vi "Axe_card.vi"(7 "Operate Axis":T1(radio), 8 "error in (no error)":errorcluster, 9 "Servo On":bool, 10 "CFG_AxJogPAssign":u32, 11 "Function":T2(ring)) -> (0 "error out":errorcluster, 1 "Axis State:":string, 2 "Position":dbl, 3 "JOGSuccess":bool)   [LabVIEW 2016]
panel:
  out "ORG":bool
  out "EZ":bool
  out "HLMT+":bool
  out "HLMT-":bool
  in  "JDec":dbl=10000.0
  in  "JAcc":dbl=10000.0
  in  "JVelL":dbl=10000.0
  in  "JVelH":dbl=10000.0
  in  "JVLTime":u32=10000
  out "Servo_Off":bool
  out "Servo_On":bool
  out "CloseSuccess":bool
  out "ResetCounter":bool
  out "StopExtDriveSuccess":bool
  out "DeviceOpened":bool
  out "AxisOpened":bool
  out "AxisHandle_Array":u32[](array[numeric])
  out "DevAxesCount":u32
  out "DeviceHandle":u32
  in  "Device Type":u16(ring)
  out "DeviceNum List":u32[](array[numeric])
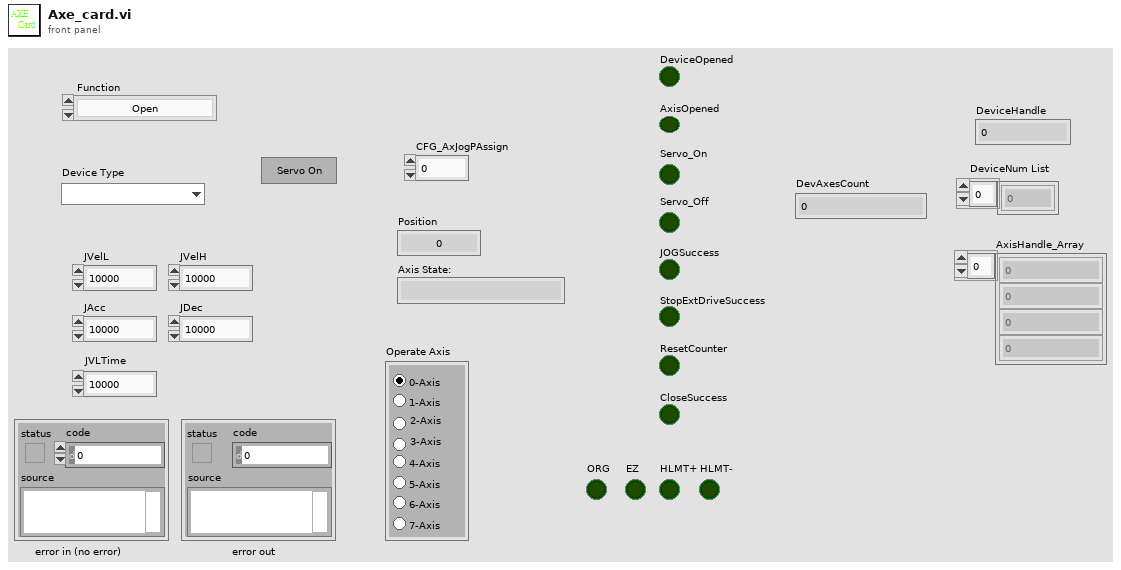
[diagram p1: front panel]
types:
  T1 = enum32{"0-Axis", "1-Axis", "2-Axis", "3-Axis", "4-Axis", "5-Axis", "6-Axis", "7-Axis"}
  T2 = enum16{"Open", "Move", "Check done", "E.Stop", "Get posion", "Home", "Serv ON/OFF", "Reset Error", "Set Param", "Close"}
  T3 = enum32{"CFG_AxJogVLTime", "CFG_AxPulseOutReverse", "CFG_AxKillDec", "CFG_AxJogVelLow", "CFG_AxJogVelHigh", "CFG_AxJogAcc", "CFG_AxJogDec", "CFG_AxJogJerk", "CFG_AxMaxErrorCnt", "CFG_AxCounterMax", "CFG_AxOverflowMode", "CFG_AxGantryActDiffValue", "CFG_AxJogPAssign", "CFG_AxJogNAssign", "CFG_AxCamDOAssign", "CFG_AxIN1StopAssign"}
  T4 = cluster{"DeviceNum":u32, "U*8 Array":cluster{"U*8 Array[0]":u8, "U*8 Array[1]":u8, "U*8 Array[2]":u8, "U*8 Array[3]":u8, "U*8 Array[4]":u8, "U*8 Array[5]":u8, "U*8 Array[6]":u8, "U*8 Array[7]":u8, "U*8 Array[8]":u8, "U*8 Array[9]":u8, "U*8 Array[10]":u8, "U*8 Array[11]":u8, "U*8 Array[12]":u8, "U*8 Array[13]":u8, "U*8 Array[14]":u8, "U*8 Array[15]":u8, "U*8 Array[16]":u8, "U*8 Array[17]":u8, "U*8 Array[18]":u8, "U*8 Array[19]":u8, "U*8 Array[20]":u8, "U*8 Array[21]":u8, "U*8 Array[22]":u8, "U*8 Array[23]":u8, "U*8 Array[24]":u8, "U*8 Array[25]":u8, "U*8 Array[26]":u8, "U*8 Array[27]":u8, "U*8 Array[28]":u8, "U*8 Array[29]":u8, "U*8 Array[30]":u8, "U*8 Array[31]":u8, "U*8 Array[32]":u8, "U*8 Array[33]":u8, "U*8 Array[34]":u8, "U*8 Array[35]":u8, "U*8 Array[36]":u8, "U*8 Array[37]":u8, "U*8 Array[38]":u8, "U*8 Array[39]":u8, "U*8 Array[40]":u8, "U*8 Array[41]":u8, "U*8 Array[42]":u8, "U*8 Array[43]":u8, "U*8 Array[44]":u8, "U*8 Array[45]":u8, "U*8 Array[46]":u8, "U*8 Array[47]":u8, "U*8 Array[48]":u8, "U*8 Array[49]":u8}, "NumOfSubDevice":i16}[]
  T5 = cluster{"U*8 Array[0]":u8, "U*8 Array[1]":u8, "U*8 Array[2]":u8, "U*8 Array[3]":u8, "U*8 Array[4]":u8, "U*8 Array[5]":u8, "U*8 Array[6]":u8, "U*8 Array[7]":u8, "U*8 Array[8]":u8, "U*8 Array[9]":u8, "U*8 Array[10]":u8, "U*8 Array[11]":u8, "U*8 Array[12]":u8, "U*8 Array[13]":u8, "U*8 Array[14]":u8, "U*8 Array[15]":u8, "U*8 Array[16]":u8, "U*8 Array[17]":u8, "U*8 Array[18]":u8, "U*8 Array[19]":u8, "U*8 Array[20]":u8, "U*8 Array[21]":u8, "U*8 Array[22]":u8, "U*8 Array[23]":u8, "U*8 Array[24]":u8, "U*8 Array[25]":u8, "U*8 Array[26]":u8, "U*8 Array[27]":u8, "U*8 Array[28]":u8, "U*8 Array[29]":u8, "U*8 Array[30]":u8, "U*8 Array[31]":u8, "U*8 Array[32]":u8, "U*8 Array[33]":u8, "U*8 Array[34]":u8, "U*8 Array[35]":u8, "U*8 Array[36]":u8, "U*8 Array[37]":u8, "U*8 Array[38]":u8, "U*8 Array[39]":u8, "U*8 Array[40]":u8, "U*8 Array[41]":u8, "U*8 Array[42]":u8, "U*8 Array[43]":u8, "U*8 Array[44]":u8, "U*8 Array[45]":u8, "U*8 Array[46]":u8, "U*8 Array[47]":u8, "U*8 Array[48]":u8, "U*8 Array[49]":u8}
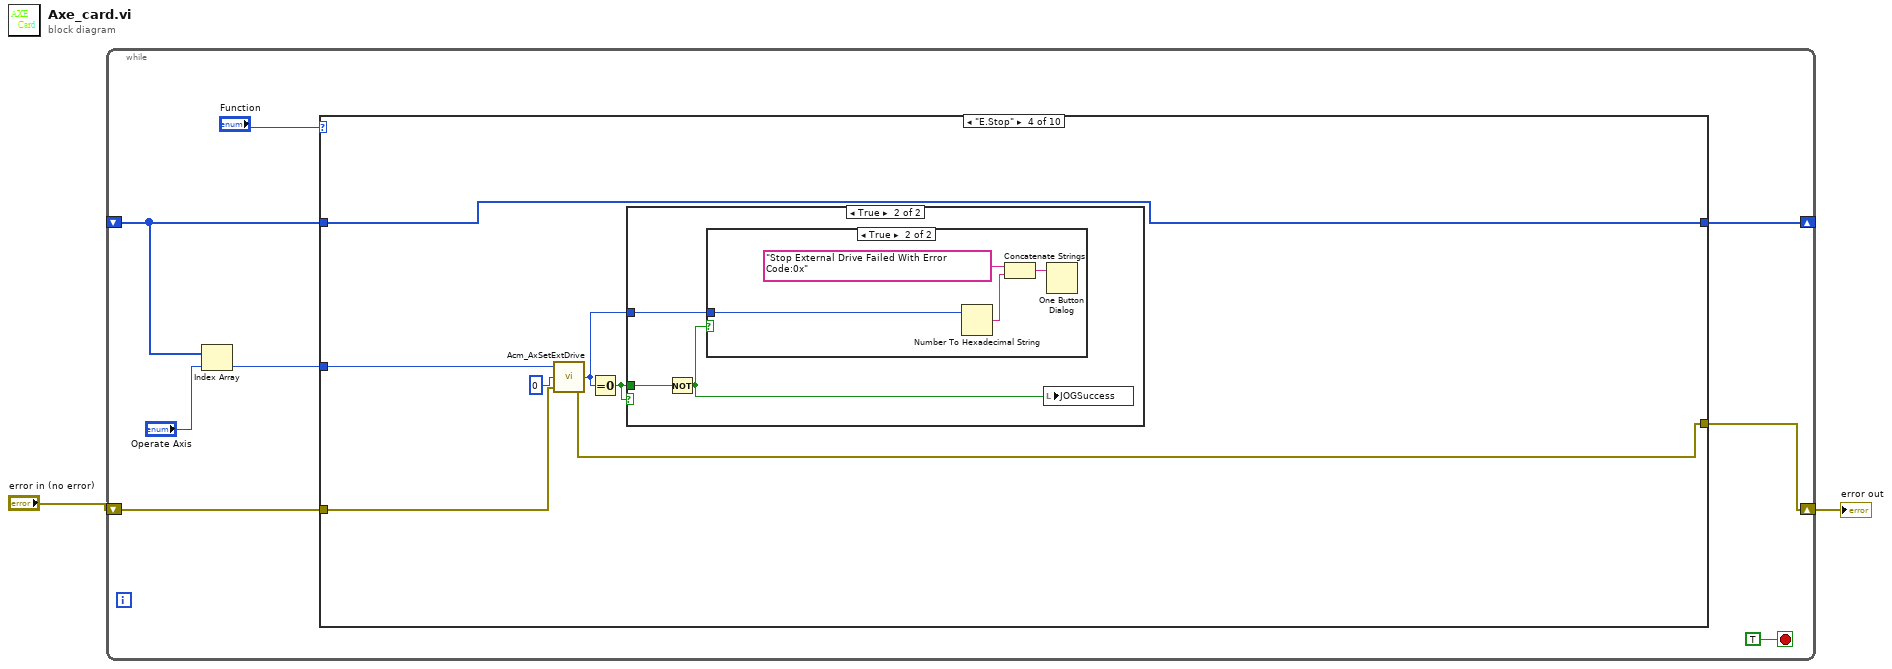
[diagram p0: block diagram]
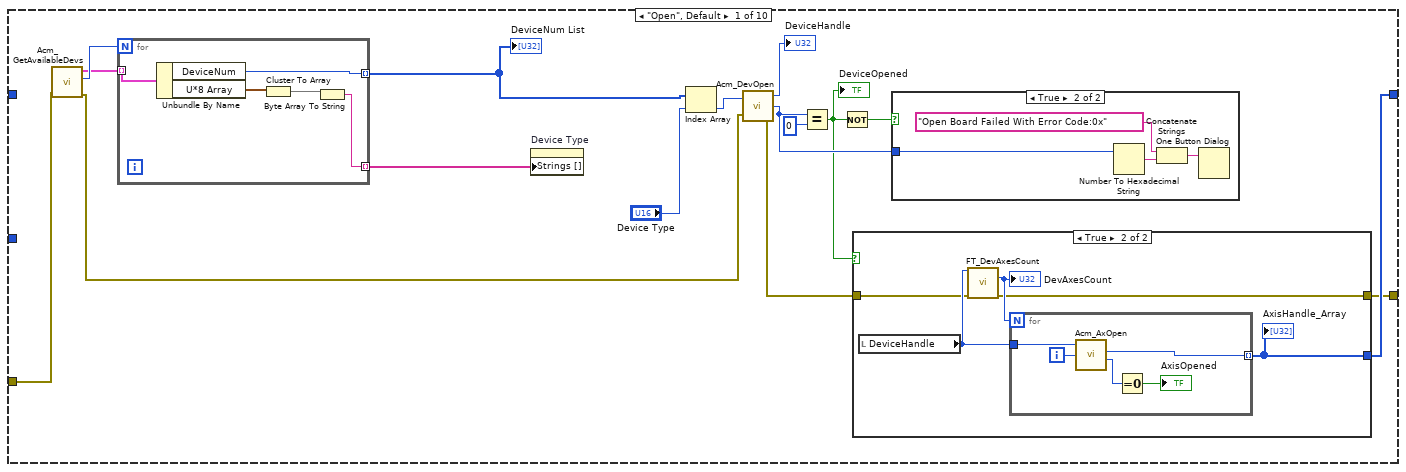
[diagram p2: hidden frame]
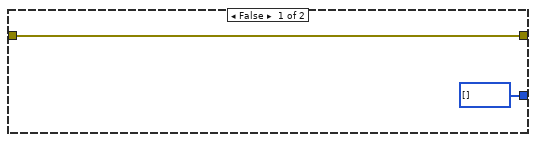
[diagram p4: hidden frame]
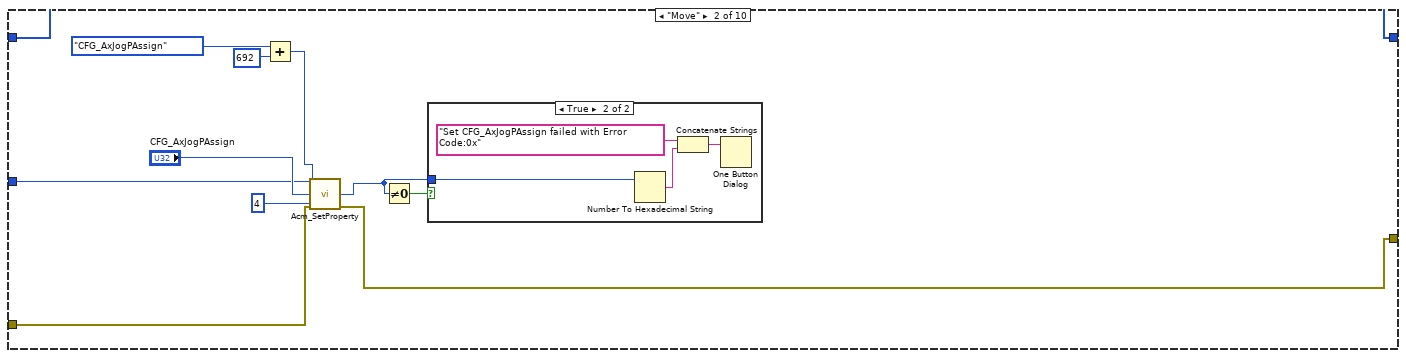
[diagram p5: hidden frame]
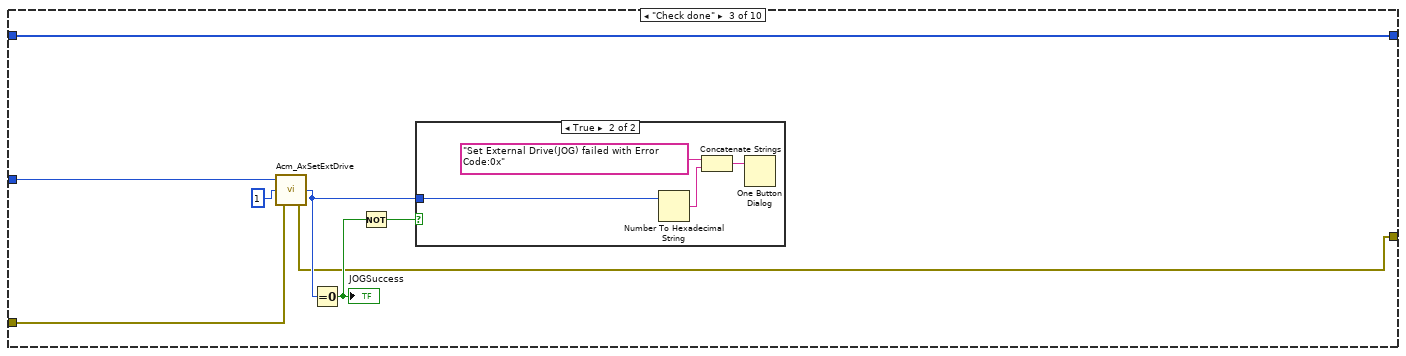
[diagram p7: hidden frame]
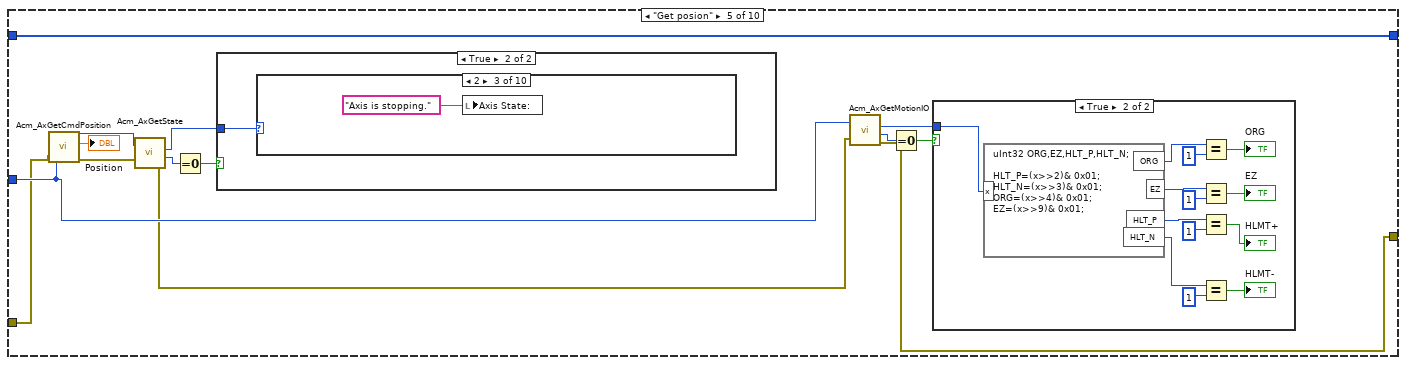
[diagram p11: hidden frame]
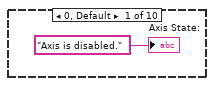
[diagram p14: hidden frame]
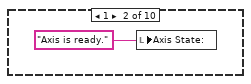
[diagram p15: hidden frame]
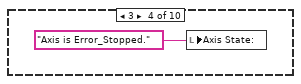
[diagram p16: hidden frame]
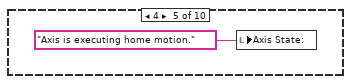
[diagram p17: hidden frame]
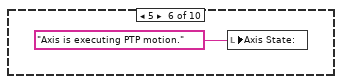
[diagram p18: hidden frame]
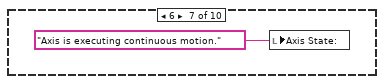
[diagram p19: hidden frame]
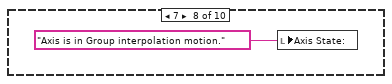
[diagram p20: hidden frame]
diagram:
  n1 = while {
    shift-right: [w8] -> _
    shift-left: _ -> [w7]
    shift-right: [w3] -> w1
    shift-left: "error in (no error)" -> [w4]
    stop <- TRUE stop-if-true
    n2 = Index Array(array=w7, index="Operate Axis") -> (element=w6:u32)
    n3 = case shown="\"E.Stop\"" "Function" {
      tunnel: [w16 w50 w65 w77 w97 w128 w149 w167 w176 w242] -> w8
      tunnel: w7 -> [_ w50 w65 w77 w97 w128 w149 w167 w176 w242]
      tunnel: w6 -> [_ w51 w66 w78 w93 w131 w151 w168 w177 _]
      tunnel: w4 -> [w14 w49 w64 w76 w92 w127 w145 w166 w175 w241]
      tunnel: [w11 w48 w63 w75 w89 w126 w144 w165 w174 w240] -> w3
      frame "Open", Default {
        n4 = call <userlib>:"Acm_GetAvailableDevs.vi"("error in (no error)"=w14) -> ("DeviceList"=w25:T4, "OutEntries"=w26:u32, "error out"=w13:errorcluster)  [unwired: 3 out]
        n5 = for {
          N: w26 -> [_]
          tunnel: w25 -> [w47] mode=indexing
          tunnel: [w44] -> w17 mode=indexing
          tunnel: [w43] -> w24 mode=indexing
          n6 = Unbundle By Name(w47) -> ("DeviceNum"=w44:u32, "U*8 Array"=w46:T5)
          n7 = Cluster To Array(cluster=w46) -> (array=w45:u8[])
          n8 = Byte Array To String(unsigned byte array=w45) -> (string=w43:string)
        }
        "DeviceNum List" <- w17
        n9 = property on="Device Type" class="Ring (strict)"("Strings []"=w24) -> ()  [unwired: 2 in, 2 out]
        n10 = Index Array(array=w17, index="Device Type") -> (element=w23:u32)
        n11 = call <userlib>:"Acm_DevOpen.vi"("error in (no error)"=w13, "DeviceNumber"=w23) -> ("error out"=w12:errorcluster, "ReturnValue"=w21:u32, "DeviceHandle"=→"DeviceHandle":u32)
        n12 = Equal?(x=w21, y=u32 0) -> (x = y?=w20:bool)
        "DeviceOpened" <- w20
        n13 = Not(x=w20) -> (.not. x?=w22:bool)
        n14 = case shown="True" w20 {
          tunnel: [u32[] [] w35] -> w16
          tunnel: w12 -> [w31 w34]
          tunnel: [w31 w33] -> w11
          frame False {
          }
          frame True {
            n15 = local read "DeviceHandle"() -> (w36:u32)
            n16 = call <userlib>:"FT_DevAxesCount.vi"("Handle"=w36, "error in (no error)"=w34) -> ("DevAxesCount"=w37:u32, "error out"=w33:errorcluster)  [unwired: 12 out]
            "DevAxesCount" <- w37
            n17 = for {
              N: w37 -> [_]
              tunnel: w36 -> [w42]
              tunnel: [w38] -> w35 mode=indexing
              i -> [w41]
              n18 = call <userlib>:"Acm_AxOpen.vi"("PhyAxis"=w41, "DeviceHandle"=w42) -> ("ReturnValue"=w40:u32, "AxisHandle"=w38:u32)  [unwired: 1 in, 2 out]
              n19 = Equal To 0?(x=w40) -> (x = 0?=→"AxisOpened":bool)
            }
            "AxisHandle_Array" <- w35
          }
        }
        n20 = case shown="True" w22 {
          tunnel: w21 -> [_ w30]
          frame False {
          }
          frame True {
            n21 = Number To Hexadecimal String(2:w30) -> (0:w28:string)  [unwired: 1 out]
            n22 = Concatenate Strings("Open Board Failed With Error Code:0x", w28) -> (w27:string)
            n23 = One Button Dialog(message=w27) -> ()  [unwired: 2 out]
          }
        }
      }
      frame "Move" {
        n24 = Add(x=T3."CFG_AxJogPAssign", y=u32 692) -> (x+y=w54:u32)
        n25 = call <userlib>:"Acm_SetProperty.vi"("Handle"=w51, "ProperyID"=w54, "Buffer"="CFG_AxJogPAssign", "BufferLength"=u32 4, "error in (no error)"=w49) -> ("ReturnValue"=w52:u32, "error out"=w48:errorcluster)  [unwired: 9 out]
        n26 = Not Equal To 0?(x=w52) -> (x != 0?=w53:bool)
        n27 = case shown="True" w53 {
          tunnel: w52 -> [_ w59]
          frame False {
          }
          frame True {
            n28 = Number To Hexadecimal String(2:w59) -> (0:w61:string)  [unwired: 1 out]
            n29 = Concatenate Strings("Set CFG_AxJogPAssign failed with Error Code:0x", w61) -> (w60:string)
            n30 = One Button Dialog(message=w60) -> ()  [unwired: 2 out]
          }
        }
      }
      frame "Check done" {
        n31 = call <userlib>:"Acm_AxSetExtDrive.vi"("error in (no error)"=w64, "ExtDrvMode"=u16 1 ("Direction"), "AxisHandle"=w66) -> ("error out"=w63:errorcluster, "ReturnValue"=w68:u32)  [unwired: 1 out]
        n32 = Equal To 0?(x=w68) -> (x = 0?=w69:bool)
        "JOGSuccess" <- w69
        n33 = Not(x=w69) -> (.not. x?=w70:bool)
        n34 = case shown="True" w70 {
          tunnel: w68 -> [_ w71]
          frame False {
          }
          frame True {
            n35 = Number To Hexadecimal String(2:w71) -> (0:w73:string)  [unwired: 1 out]
            n36 = Concatenate Strings("Set External Drive(JOG) failed with Error Code:0x", w73) -> (w72:string)
            n37 = One Button Dialog(message=w72) -> ()  [unwired: 2 out]
          }
        }
      }
      frame "E.Stop" {
        n38 = call <userlib>:"Acm_AxSetExtDrive.vi"("error in (no error)"=w76, "ExtDrvMode"=u16 0, "AxisHandle"=w78) -> ("error out"=w75:errorcluster, "ReturnValue"=w81:u32)  [unwired: 1 out]
        n39 = Equal To 0?(x=w81) -> (x = 0?=w79:bool)
        n40 = case shown="True" w79 {
          tunnel: w81 -> [_ w84]
          tunnel: w79 -> [_ w83]
          frame False {
          }
          frame True {
            n41 = Not(x=w83) -> (.not. x?=w82:bool)
            n42 = case shown="True" w82 {
              tunnel: w84 -> [_ w88]
              frame False {
              }
              frame True {
                n43 = Number To Hexadecimal String(2:w88) -> (0:w86:string)  [unwired: 1 out]
                n44 = Concatenate Strings("Stop External Drive Failed With Error Code:0x", w86) -> (w85:string)
                n45 = One Button Dialog(message=w85) -> ()  [unwired: 2 out]
              }
            }
            n46 = local write "JOGSuccess"(w82) -> ()
          }
        }
      }
      frame "Get posion" {
        n47 = call <userlib>:"Acm_AxGetCmdPosition.vi"("error in (no error)"=w92, "AxisHandle"=w93) -> ("error out"=w91:errorcluster, "Position"=→"Position":dbl)  [unwired: 2 out]
        n48 = call <userlib>:"Acm_AxGetState.vi"("error in (no error)"=w91, "AxisHandle"=w93) -> ("error out"=w90:errorcluster, "ReturnValue"=w98:u32, "Status"=w100:u16)  [unwired: 1 out]
        n49 = Equal To 0?(x=w98) -> (x = 0?=w99:bool)
        n50 = case shown="True" w99 {
          tunnel: w100 -> [_ w115]
          frame False {
          }
          frame True {
            n51 = case shown="2" w115 {
              frame 0, Default {
                "Axis State:" <- "Axis is disabled." ("Axis State:")
              }
              frame 1 {
                n52 = local write "Axis State:"("Axis is ready." ("Axis State:")) -> ()
              }
              frame 2 {
                n53 = local write "Axis State:"("Axis is stopping." ("Axis State:")) -> ()
              }
              frame 3 {
                n54 = local write "Axis State:"("Axis is Error_Stopped." ("Axis State:")) -> ()
              }
              frame 4 {
                n55 = local write "Axis State:"("Axis is executing home motion." ("Axis State:")) -> ()
              }
              frame 5 {
                n56 = local write "Axis State:"("Axis is executing PTP motion." ("Axis State:")) -> ()
              }
              frame 6 {
                n57 = local write "Axis State:"("Axis is executing continuous motion." ("Axis State:")) -> ()
              }
              frame 7 {
                n58 = local write "Axis State:"("Axis is in Group interpolation motion." ("Axis State:")) -> ()
              }
              frame 8 {
                n59 = local write "Axis State:"("Axis is executing JOG mode motion." ("Axis State:")) -> ()
              }
              frame 9 {
                n60 = local write "Axis State:"("Axis is executing MPG mode motion." ("Axis State:")) -> ()
              }
            }
          }
        }
        n61 = call <userlib>:"Acm_AxGetMotionIO.vi"("error in (no error)"=w90, "AxisHandle"=w93) -> ("error out"=w89:errorcluster, "ReturnValue"=w94:u32, "Status"=w96:u32)  [unwired: 1 out]
        n62 = Equal To 0?(x=w94) -> (x = 0?=w95:bool)
        n63 = case shown="True" w95 {
          tunnel: w96 -> [_ w114]
          frame False {
          }
          frame True {
            n64 = formula code="uInt32 ORG,EZ,HLT_P,HLT_N;\n\nHLT_P=(x>>2)& 0x01;\nHLT_N=(x>>3)& 0x01;\nORG=(x>>4)& 0x01;\nEZ=(x>>9)& 0x01;"("x"=w114) -> ("ORG"=w112:u32, "EZ"=w110:u32, "HLT_P"=w108:u32, "HLT_N"=w103:u32)
            n65 = Equal?(x=w112, y=u32 1) -> (x = y?=→"ORG":bool)
            n66 = Equal?(x=w110, y=u32 1) -> (x = y?=→"EZ":bool)
            n67 = Equal?(x=w108, y=u32 1) -> (x = y?=→"HLMT+":bool)
            n68 = Equal?(x=w103, y=u32 1) -> (x = y?=→"HLMT-":bool)
          }
        }
      }
      frame "Serv ON/OFF" {
        n69 = Boolean To (0,1)(Boolean="Servo On") -> (0, 1=w130:i16)
        n70 = call <userlib>:"Acm_AxSetSvOn.vi"("error in (no error)"=w127, "OnOff"=w130, "AxisHandle"=w131) -> ("error out"=w126:errorcluster, "ReturnValue"=w135:u32)  [unwired: 1 out]
        n71 = Not Equal To 0?(x=w135) -> (x != 0?=w132:bool)
        n72 = Not(x=w132) -> (.not. x?=w133:bool)
        n73 = case shown="True" w132 {
          tunnel: w135 -> [_ w140]
          frame False {
          }
          frame True {
            w143 = "Servo On/Off Failed With Error Code:0x"  # Servo On/Off Failed With Error Code:0x
            n74 = Number To Hexadecimal String(2:w140) -> (0:w142:string)  [unwired: 1 out]
            n75 = Concatenate Strings(w143, w142) -> (w141:string)
            n76 = One Button Dialog(message=w141) -> ()  [unwired: 2 out]
          }
        }
        n77 = And(x="Servo On", y=w133) -> (x .and. y?=w134:bool)
        n78 = case shown="True" w134 {
          frame False {
            "Servo_On" <- FALSE ("Servo_On")
            "Servo_Off" <- TRUE ("Servo_Off")
          }
          frame True {
            n79 = local write "Servo_Off"(TRUE ("Servo_On")) -> ()
            n80 = local write "Servo On"(FALSE ("Servo_Off")) -> ()
          }
        }
      }
      frame "Home" {
        n81 = Add(x=T3."CFG_AxJogPAssign", y=u32 692) -> (x+y=w157:u32)
        n82 = call <userlib>:"Acm_SetProperty.vi"("Handle"=w151, "ProperyID"=w157, "Buffer"=u32 100000, "BufferLength"=u32 4, "error in (no error)"=w145) -> ("ReturnValue"=w155:u32, "error out"=w146:errorcluster)  [unwired: 9 out]
        n83 = Not Equal To 0?(x=w155) -> (x != 0?=w156:bool)
        n84 = call <userlib>:"Acm_AxSetExtDrive.vi"("error in (no error)"=w146, "ExtDrvMode"=u16 1 ("Direction")) -> ("ReturnValue"=w148:u32)  [unwired: 1 in, 2 out]
        n85 = case shown="True" w156 {
          tunnel: w155 -> [_ w161]
          frame False {
          }
          frame True {
            n86 = Number To Hexadecimal String(2:w161) -> (0:w163:string)  [unwired: 1 out]
            n87 = Concatenate Strings("Set CFG_AxJogPAssign failed with Error Code:0x", w163) -> (w162:string)
            n88 = One Button Dialog(message=w162) -> ()  [unwired: 2 out]
          }
        }
        n89 = Equal To 0?(x=w148) -> ()  [unwired: 1 out]
        n90 = call <userlib>:"Acm_AxSetCmdPosition.vi"("error in (no error)"=w146, "Position"=0.0, "AxisHandle"=w151) -> ("error out"=w144:errorcluster, "ReturnValue"=w152:u32)  [unwired: 1 out]
        n91 = Equal To 0?(x=w152) -> (x = 0?=→"ResetCounter":bool)
      }
      frame "Reset Error" {
        n92 = local read "AxisOpened"() -> (w169:bool)
        n93 = case shown="False" w169 {
          tunnel: w168 -> [_ w173]
          tunnel: w166 -> [w170 w172]
          tunnel: [w170 w171] -> w165
          frame False {
          }
          frame True {
            n94 = call <userlib>:"Acm_AxResetError.vi"("error in (no error)"=w172, "AxisHandle"=w173) -> ("error out"=w171:errorcluster)  [unwired: 2 out]
          }
        }
      }
      frame "Set Param" {
        n95 = stacked-sequence {
          tunnel: w177 -> [w182 w193 w205 w217 w230]
          tunnel: w175 -> [w179 _ _ _ _]
          tunnel: [w178 _ _ _ _] -> w174
          frame #0 {
            n96 = Add(x=T3."CFG_AxJogVLTime", y=u32 692) -> (x+y=w183:u32)
            n97 = call <userlib>:"Acm_SetProperty.vi"("Handle"=w182, "ProperyID"=w183, "Buffer"="JVLTime", "BufferLength"=u32 4, "error in (no error)"=w179) -> ("ReturnValue"=w181:u32, "error out"=w178:errorcluster)  [unwired: 9 out]
            n98 = Not Equal To 0?(x=w181) -> (x != 0?=w187:bool)
            n99 = case shown="True" w187 {
              tunnel: w181 -> [_ w188]
              frame False {
              }
              frame True {
                n100 = Number To Hexadecimal String(2:w188) -> (0:w190:string)  [unwired: 1 out]
                n101 = Concatenate Strings("Set CFG_AxJogVLTime failed with Error Code:0x", w190) -> (w189:string)
                n102 = One Button Dialog(message=w189) -> ()  [unwired: 2 out]
              }
            }
          }
          frame #1 {
            n103 = Add(x=T3."CFG_AxJogVelHigh", y=u32 692) -> (x+y=w195:u32)
            n104 = call <userlib>:"Acm_SetProperty.vi"("Handle"=w193, "ProperyID"=w195, "Buffer"="JVelH", "BufferLength"=u32 8) -> ("ReturnValue"=w192:u32)  [unwired: 1 in, 10 out]
            n105 = Not Equal To 0?(x=w192) -> (x != 0?=w199:bool)
            n106 = case shown="True" w199 {
              tunnel: w192 -> [_ w200]
              frame False {
              }
              frame True {
                n107 = Number To Hexadecimal String(2:w200) -> (0:w202:string)  [unwired: 1 out]
                n108 = Concatenate Strings("Set CFG_AxJogVelHigh failed with Error Code:0x", w202) -> (w201:string)
                n109 = One Button Dialog(message=w201) -> ()  [unwired: 2 out]
              }
            }
          }
          frame #2 {
            n110 = Add(x=T3."CFG_AxJogVelLow", y=u32 692) -> (x+y=w207:u32)
            n111 = call <userlib>:"Acm_SetProperty.vi"("Handle"=w205, "ProperyID"=w207, "Buffer"="JVelL", "BufferLength"=u32 8) -> ("ReturnValue"=w204:u32)  [unwired: 1 in, 10 out]
            n112 = Not Equal To 0?(x=w204) -> (x != 0?=w211:bool)
            n113 = case shown="True" w211 {
              tunnel: w204 -> [_ w212]
              frame False {
              }
              frame True {
                n114 = Number To Hexadecimal String(2:w212) -> (0:w214:string)  [unwired: 1 out]
                n115 = Concatenate Strings("Set CFG_AxJogVelLow failed with Error Code:0x", w214) -> (w213:string)
                n116 = One Button Dialog(message=w213) -> ()  [unwired: 2 out]
              }
            }
          }
          frame #3 {
            n117 = Add(x=T3."CFG_AxJogAcc", y=u32 692) -> (x+y=w220:u32)
            n118 = call <userlib>:"Acm_SetProperty.vi"("Handle"=w217, "ProperyID"=w220, "Buffer"="JAcc", "BufferLength"=u32 8) -> ("ReturnValue"=w218:u32)  [unwired: 1 in, 10 out]
            n119 = Not Equal To 0?(x=w218) -> (x != 0?=w223:bool)
            n120 = case shown="True" w223 {
              tunnel: w218 -> [_ w224]
              frame False {
              }
              frame True {
                n121 = Number To Hexadecimal String(2:w224) -> (0:w226:string)  [unwired: 1 out]
                n122 = Concatenate Strings("Set CFG_AxJogAcc failed with Error Code:0x", w226) -> (w225:string)
                n123 = One Button Dialog(message=w225) -> ()  [unwired: 2 out]
              }
            }
          }
          frame #4 {
            n124 = Add(x=T3."CFG_AxJogDec", y=u32 692) -> (x+y=w231:u32)
            n125 = call <userlib>:"Acm_SetProperty.vi"("Handle"=w230, "ProperyID"=w231, "Buffer"="JDec", "BufferLength"=u32 8) -> ("ReturnValue"=w229:u32)  [unwired: 1 in, 10 out]
            n126 = Not Equal To 0?(x=w229) -> (x != 0?=w235:bool)
            n127 = case shown="True" w235 {
              tunnel: w229 -> [_ w236]
              frame False {
              }
              frame True {
                n128 = Number To Hexadecimal String(2:w236) -> (0:w238:string)  [unwired: 1 out]
                n129 = Concatenate Strings("Set CFG_AxJogDec failed with Error Code:0x", w238) -> (w237:string)
                n130 = One Button Dialog(message=w237) -> ()  [unwired: 2 out]
              }
            }
          }
        }
      }
      frame "Close" {
        n131 = stacked-sequence {
          tunnel: w241 -> [_ w251]
          tunnel: [_ w250] -> w240
          frame #0 {
            n132 = local read "DevAxesCount"() -> (w243:u32)
            n133 = for {
              N: w243 -> [_]
              i -> [w248]
              n134 = local read "AxisHandle_Array"() -> (w249:u32[])
              n135 = Index Array(array=w249, index=w248) -> (element=w247:u32)
              n136 = call <userlib>:"Acm_AxClose.vi"("AxisHandle"=w247) -> ("ReturnValue"=w246:u32)  [unwired: 1 in, 1 out]
              n137 = Equal To 0?(x=w246) -> (x = 0?=w245:bool)
              n138 = Not(x=w245) -> (.not. x?=w244:bool)
              n139 = local write "AxisOpened"(w244) -> ()
            }
          }
          frame #1 {
            n140 = local read "DeviceHandle"() -> (w255:u32)
            n141 = call <userlib>:"Acm_DevClose.vi"("error in (no error)"=w251, "DeviceHandle"=w255) -> ("error out"=w250:errorcluster, "ReturnValue"=w253:u32)  [unwired: 2 out]
            n142 = Equal To 0?(x=w253) -> (x = 0?=w252:bool)
            "CloseSuccess" <- w252
            n143 = Not(x=w252) -> (.not. x?=w254:bool)
            n144 = case shown="True" w252 {
              tunnel: w252 -> [_ w265]
              frame False {
              }
              frame True {
                n145 = Not(x=w265) -> (.not. x?=w260:bool)
                "StopExtDriveSuccess" <- w260
                n146 = local write "DevAxesCount"(u32 0 ("DevAxesCount")) -> ()
                n147 = local write "DeviceHandle"(u32 0 ("DeviceHandle")) -> ()
                n148 = local read "DevAxesCount"() -> (w262:u32)
                n149 = local write "ResetCounter"(w260) -> ()
                n150 = Initialize Array(u32 0 ("元素"), w262) -> (w263:u32[])
                n151 = local write "AxisHandle_Array"(w263) -> ()
              }
            }
            n152 = case shown="True" w254 {
              tunnel: w253 -> [_ w256]
              frame False {
              }
              frame True {
                n153 = Number To Hexadecimal String(2:w256) -> (0:w258:string)  [unwired: 1 out]
                n154 = Concatenate Strings("Close Board Failed With Error Code:0x", w258) -> (w257:string)
                n155 = One Button Dialog(message=w257) -> ()  [unwired: 2 out]
              }
            }
          }
        }
      }
    }
  }
  "error out" <- w1
